vi "ReadFullScaleRangePressure Example.vi"() -> ()   [LabVIEW 2019]
uses:
  BrooksDLL.dll
panel:
  out "PressureUnit String":string
  out "FullScalePressure":sgl format="%.2f"
  out "Pressure Unit Code":u8
  in  "Pressure Application":u8=1 min=1 max=6 step=1
  out "S2 String":string
  out "S1 String":string
  out "S2":u8 format="%.0x"
  out "S1":u8 format="%.0x"
  out "Function Output Comment":string
  out "output param":i32
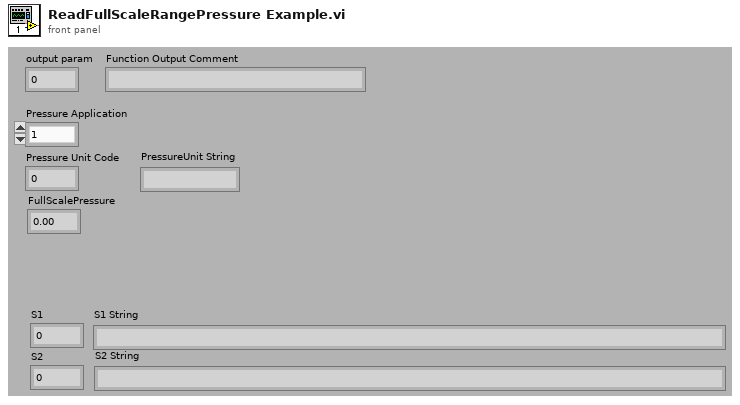
[diagram p1: front panel]
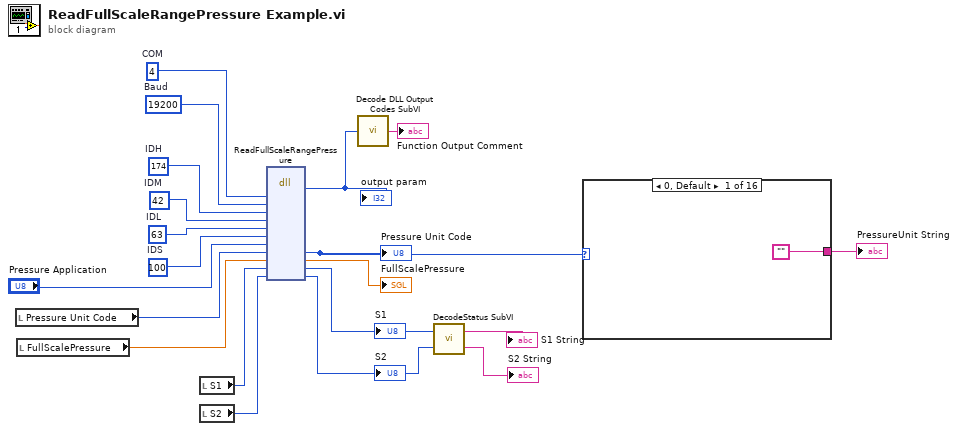
[diagram p0: block diagram]
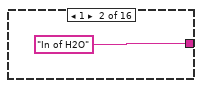
[diagram p2: hidden frame]
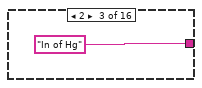
[diagram p3: hidden frame]
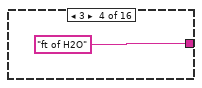
[diagram p4: hidden frame]
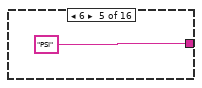
[diagram p5: hidden frame]
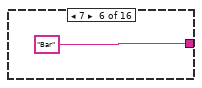
[diagram p6: hidden frame]
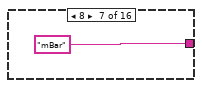
[diagram p7: hidden frame]
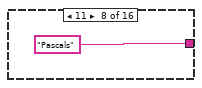
[diagram p8: hidden frame]
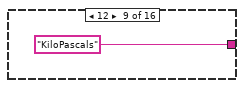
[diagram p9: hidden frame]
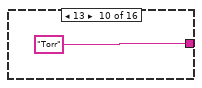
[diagram p10: hidden frame]
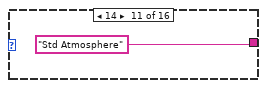
[diagram p11: hidden frame]
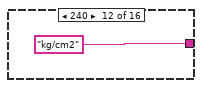
[diagram p12: hidden frame]
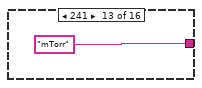
[diagram p13: hidden frame]
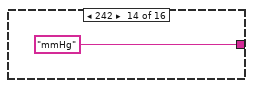
[diagram p14: hidden frame]
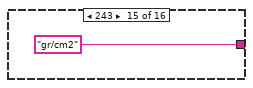
[diagram p15: hidden frame]
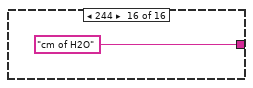
[diagram p16: hidden frame]
diagram:
  w15 = u8 100  # IDS
  w16 = u8 63  # IDL
  w17 = u8 42  # IDM
  w18 = u8 174  # IDH
  w19 = 19200  # Baud
  w20 = 4  # COM
  n1 = local read "Pressure Unit Code"() -> (w10:u8)
  n2 = local read "FullScalePressure"() -> (w6:sgl)
  n3 = local read "S1"() -> (w5:u8)
  n4 = local read "S2"() -> (w4:u8)
  n5 = dll-call lib="G:/Developpement_de_Programmes/Programmes/Controle de pression/164J027_AD/Brooks DLL 1.0.1.0 32bit/Brooks DLL 1.0.1.0 Release 10032016/S Protocol/BrooksDLL.dll" fn="ReadFullScaleRangePressure"("COM"=w20, "Baud"=w19, "IDH"=w18, "IDM"=w17, "IDL"=w16, "IDS"=w15, "PressureApplication"="Pressure Application", "PressureUnitCode"=w10, "FullScalePressure"=w6, "S1"=w5, "S2"=w4) -> (w14:i32, "PressureUnitCode"=w8:u8, "FullScalePressure"=→"FullScalePressure":sgl, "S1"=w3:u8, "S2"=w2:u8)  [unwired: 10 in, 2 out]
  "output param" <- w14
  "S1" <- w3
  "S2" <- w2
  "Pressure Unit Code" <- w8
  n6 = call "Decode DLL Output Codes SubVI.vi"("Numeric"=w14) -> ("Function Output Comment"=→"Function Output Comment":string)
  n7 = call "DecodeStatus SubVI.vi"("S2"=w2, "S1"=w3) -> ("S2 String"=→"S2 String":string, "S1 String"=→"S1 String":string)
  n8 = case shown="0, Default" w8 {
    tunnel: ["" "In of H2O" "In of Hg" "ft of H2O" "PSI" "Bar" "mBar" "Pascals" "KiloPascals" "Torr" "Std Atmosphere" "kg/cm2" "mTorr" "mmHg" "gr/cm2" "cm of H2O"] -> w1
    frame 0, Default {
    }
    frame 1 {
    }
    frame 2 {
    }
    frame 3 {
    }
    frame 6 {
    }
    frame 7 {
    }
    frame 8 {
    }
    frame 11 {
    }
    frame 12 {
    }
    frame 13 {
    }
    frame 14 {
    }
    frame 240 {
    }
    frame 241 {
    }
    frame 242 {
    }
    frame 243 {
    }
    frame 244 {
    }
  }
  "PressureUnit String" <- w1
